vi "Get File Name.vi"(8 "Error In":errorcluster, 10 "Module Init Timestamp":timestamp, 11 "Application Name":string) -> (0 "Error Out":errorcluster, 3 "Error Log Filename":string)   [LabVIEW 2016, in "Error Manager.lvlib" / "Error Log.lvclass"]
uses:
  Error Log.lvclass
panel:
  out "Timestamp String":string
  # "Input\nInputs to the VI"
  # "Development\nControls or indicators that are useful for development or testing, but which are not outputs of the VI."
  # "Output\nOutputs of the VI"
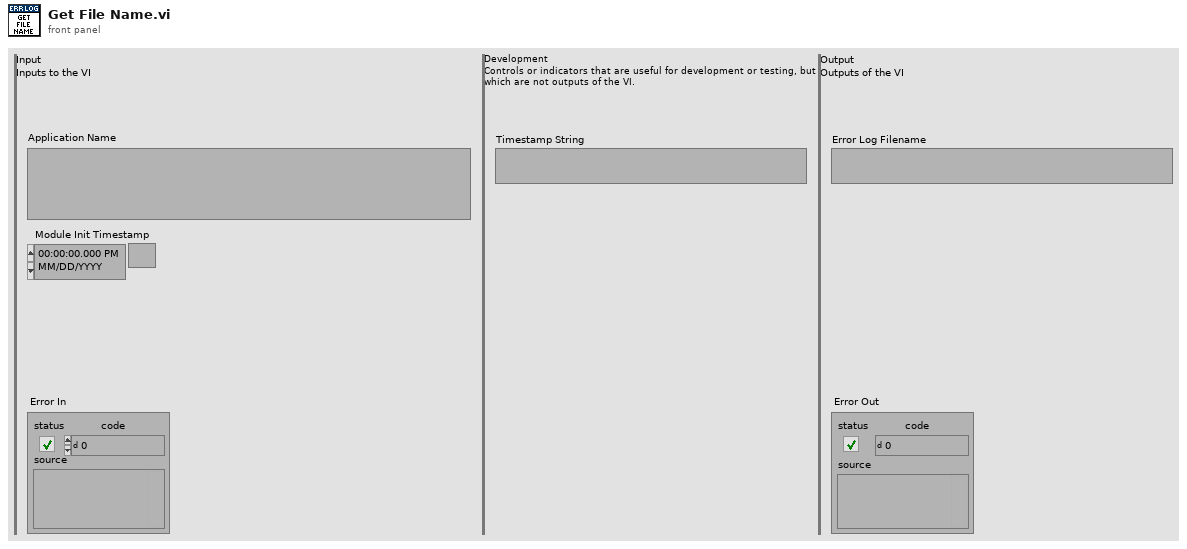
[diagram p1: front panel]
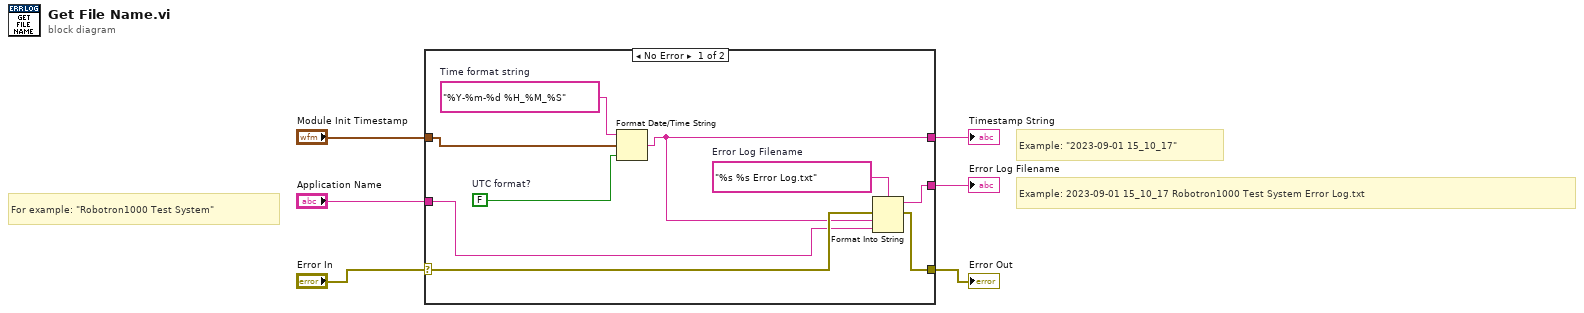
[diagram p0: block diagram]
diagram:
  # "Example: \"2023-09-01 15_10_17\""
  # "For example: \"Robotron1000 Test System\""
  # "Example: 2023-09-01 15_10_17 Robotron1000 Test System Error Log.txt"
  n1 = case shown="No Error" "Error In" {
    selector: "Error In" -> [w13 w16]
    tunnel: [w12 w16] -> w5
    tunnel: [w14 _] -> w4
    tunnel: "Application Name" -> [w11 _]
    tunnel: "Module Init Timestamp" -> [w7 _]
    tunnel: [w8 _] -> w1
    frame No Error {
      w9 = "%Y-%m-%d %H_%M_%S"  # Time format string
      w10 = FALSE  # UTC format?
      w15 = "%s %s Error Log.txt"  # Error Log Filename
      n2 = Format Date/Time String(time format string (%c)=w9, seconds (now)=w7, UTC format=w10) -> (date/time string=w8:string)
      n3 = Format Into String(format string=w15, error in=w13, w8, w11) -> (resulting string=w14:string, error out=w12:errorcluster)  [unwired: 1 in]
    }
    frame Error {
    }
  }
  "Error Out" <- w5
  "Error Log Filename" <- w4
  "Timestamp String" <- w1
